vi "select requested data from MC tcp queue.vi"(10 "TCP subscriptions info":T1, 11 "All data":string[][](array[string])) -> (2 "Array":string[](array[string]), 3 "Data out":string[][](array[string]))   [LabVIEW 2020]
uses:
  Shared/GUI_Template/TCP subscription info cluster.ctl
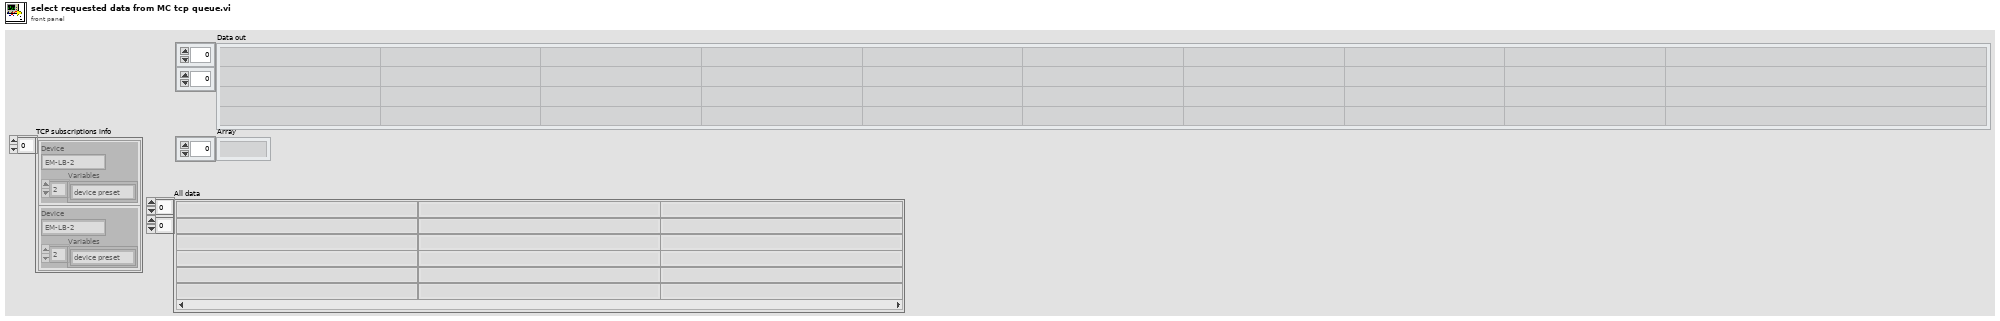
[diagram p1: front panel]
types:
  T1 = typedef "TCP subscription info cluster.ctl" = cluster{"Device":string, "Variables":string[]}[]
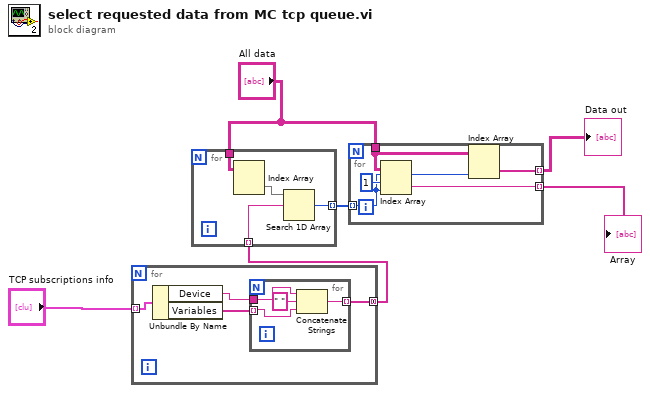
[diagram p0: block diagram]
diagram:
  n1 = for {
    tunnel: "TCP subscriptions info" -> [w10] mode=indexing
    tunnel: [w8] -> w1 mode=concatenating
    n2 = Unbundle By Name(w10) -> ("Device"=w9:string, "Variables"=w7:string[])
    n3 = for {
      tunnel: w9 -> [w13]
      tunnel: w7 -> [w12] mode=indexing
      tunnel: [w11] -> w8 mode=indexing
      n4 = Concatenate Strings(w13, " " ("string"), w12) -> (w11:string)
    }
  }
  n5 = for {
    tunnel: "All data" -> [w18]
    tunnel: w1 -> [w16] mode=indexing
    tunnel: [w15] -> w4 mode=indexing
    n6 = Index Array(array=w18) -> (element=w17:string[])  [unwired: 2 in]
    n7 = Search 1D Array(1D array=w17, element=w16) -> (index of element=w15:i32)  [unwired: 1 in]
  }
  n8 = for {
    tunnel: "All data" -> [w21]
    tunnel: w4 -> [w20] mode=indexing
    tunnel: [w22] -> w3 mode=indexing
    tunnel: [w19] -> w6 mode=indexing
    n9 = Index Array(array=w21, index (row)=1, index (col)=w20) -> (element=w22:string)
    n10 = Index Array(array=w21, index (col)=w20) -> (element=w19:string[])  [unwired: 1 in]
  }
  "Data out" <- w6
  "Array" <- w3
